vi "Sort String Array by Numeric Suffix.vi"(8 "Ignore File Extension":bool, 11 "String Array":string[](array[string])) -> (0 "Root String":string, 1 "Sorted Indices":i32[](array[numeric]), 3 "Sorted String Array":string[](array[string]))   [LabVIEW 2021, in "Strings.lvlib"]
uses:
  Strings.lvlib
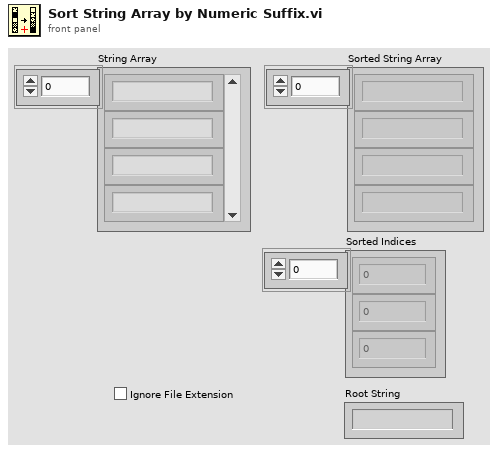
[diagram p1: front panel]
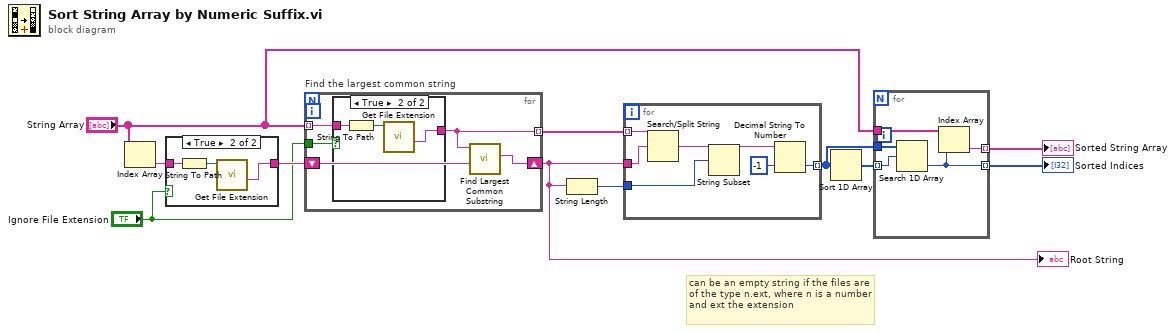
[diagram p0: block diagram]
diagram:
  # "can be an empty string if the files are of the type n.ext, where n is a number and ext the extension"
  n1 = Index Array(array="String Array") -> (element=w9:string)  [unwired: 1 in]
  n2 = case shown="True" "Ignore File Extension" {
    tunnel: w9 -> [w12 w15]
    tunnel: [w12 w13] -> w8
    frame False {
    }
    frame True {
      n3 = String To Path(string=w15) -> (path=w14:path)
      n4 = call <vilib>:"Get File Extension.vi"("file"=w14) -> ("filename without extension"=w13:string)  [unwired: 6 in, 4 out]
    }
  }
  n5 = for "Find the largest common string" {
    tunnel: "String Array" -> [w18] mode=indexing
    shift-right: [w19] -> w3
    shift-left: w8 -> [w20]
    tunnel: "Ignore File Extension" -> [w17]
    tunnel: [w16] -> w4 mode=indexing
    n6 = case shown="True" w17 {
      tunnel: w18 -> [w21 w24]
      tunnel: [w21 w22] -> w16
      frame False {
      }
      frame True {
        n7 = String To Path(string=w24) -> (path=w23:path)
        n8 = call <vilib>:"Get File Extension.vi"("file"=w23) -> ("filename without extension"=w22:string)  [unwired: 6 in, 4 out]
      }
    }
    n9 = call "Find Largest Common Substring.vi"("String 2"=w20, "String 1"=w16) -> ("Largest Common String"=w19:string)  [unwired: 7 in, 2 out]
  }
  "Root String" <- w3
  n10 = String Length(string=w3) -> (length=w2:i32)
  n11 = for {
    tunnel: w4 -> [w31] mode=indexing
    tunnel: w3 -> [w30]
    tunnel: [w29] -> w5 mode=indexing
    tunnel: w2 -> [w25]
    n12 = Search/Split String(string=w31, search string/char (-)=w30) -> (match + rest of string=w27:string)  [unwired: 1 in, 2 out]
    n13 = String Subset(string=w27, offset (0)=w25) -> (substring=w26:string)  [unwired: 1 in]
    n14 = Decimal String To Number(string=w26, default (0L)=-1 ("default (0 I32)")) -> (number=w29:i32)  [unwired: 1 in, 1 out]
  }
  n15 = Sort 1D Array(array=w5) -> (sorted array=w6:i32[])
  n16 = for {
    tunnel: w6 -> [w36] mode=indexing
    tunnel: w5 -> [w35]
    tunnel: "String Array" -> [w34]
    tunnel: [w33] -> w11 mode=indexing
    tunnel: [w32] -> w10 mode=indexing
    n17 = Search 1D Array(1D array=w35, element=w36) -> (index of element=w32:i32)  [unwired: 1 in]
    n18 = Index Array(array=w34, index=w32) -> (element=w33:string)
  }
  "Sorted String Array" <- w11
  "Sorted Indices" <- w10
